vi "Is Number Prime.vi"(10 "number":u32) -> (2 "is prime":bool)   [LabVIEW 2021]
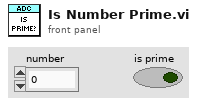
[diagram p1: front panel]
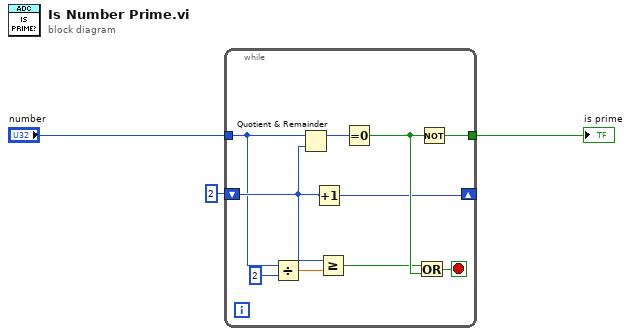
[diagram p0: block diagram]
diagram:
  n1 = while {
    shift-right: [w9] -> _
    shift-left: u32 2 -> [w8]
    tunnel: "number" -> [w5]
    tunnel: [w10] -> w3
    stop <- w12 stop-if-true
    n2 = Divide(x=w5, y=u32 2) -> (x/y=w6:dbl)
    n3 = Quotient & Remainder(x=w5, y=w8) -> (x-y*floor(x/y)=w13:u32)  [unwired: 1 out]
    n4 = Increment(x=w8) -> (x+1=w9:u32)
    n5 = Greater Or Equal?(x=w8, y=w6) -> (x >= y?=w7:bool)
    n6 = Equal To 0?(x=w13) -> (x = 0?=w11:bool)
    n7 = Or(x=w7, y=w11) -> (x .or. y?=w12:bool)
    n8 = Not(x=w11) -> (.not. x?=w10:bool)
  }
  "is prime" <- w3
